vi "cw_3_4.vi"() -> ()   [LabVIEW 2022 SP3]
panel:
  out "initialized array":i32[][](array[numeric])
  in  "M":i32
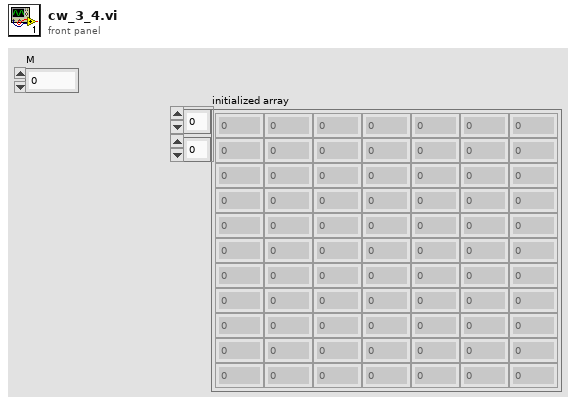
[diagram p1: front panel]
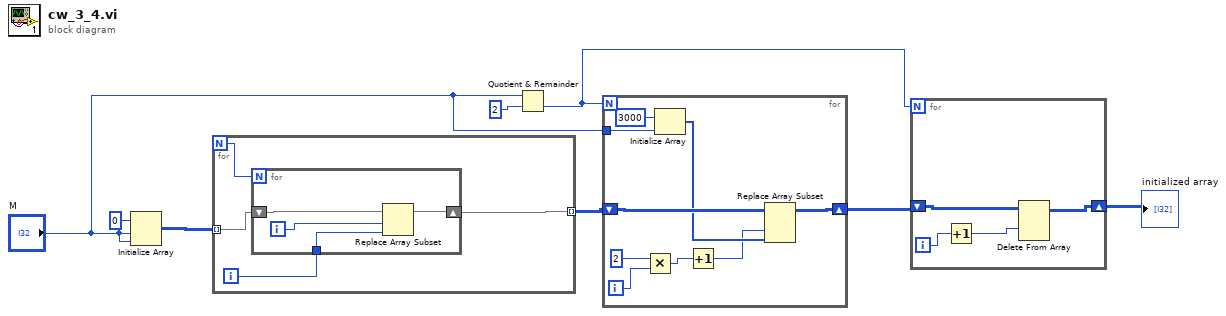
[diagram p0: block diagram]
diagram:
  n1 = Initialize Array(0 ("element"), "M", "M") -> (w7:i32[][])
  n2 = for {
    N -> [w12]
    tunnel: w7 -> [w11] mode=indexing
    tunnel: [w10] -> w4 mode=indexing
    i -> [w9]
    n3 = for {
      N: w12 -> [_]
      shift-right: [w15] -> w10
      shift-left: w11 -> [w16]
      tunnel: w9 -> [w13]
      i -> [w14]
      n4 = Replace Array Subset(array=w16, new element=w13, index=w14) -> (w15:i32[])
    }
  }
  n5 = Quotient & Remainder(x="M", y=2) -> (floor(x/y)=w3:i32)  [unwired: 1 out]
  n6 = for {
    N: w3 -> [_]
    tunnel: "M" -> [w25]
    shift-right: [w20] -> w2
    shift-left: w4 -> [w21]
    i -> [w23]
    n7 = Multiply(x=2, y=w23) -> (x*y=w18:i32)
    n8 = Initialize Array(3000 ("element"), w25) -> (w19:i32[])
    n9 = Increment(x=w18) -> (x+1=w17:i32)
    n10 = Replace Array Subset(array=w21, new element=w19, index (col)=w17) -> (w20:i32[][])  [unwired: 1 in]
  }
  n11 = for {
    N: w3 -> [_]
    shift-right: [w28] -> w1
    shift-left: w2 -> [w29]
    i -> [w27]
    n12 = Increment(x=w27) -> (x+1=w26:i32)
    n13 = Delete From Array(array=w29, index (row)=w26) -> (array with subset deleted=w28:i32[][])  [unwired: 2 in, 1 out]
  }
  "initialized array" <- w1
